vi "PixyCamSPI.vi"(11 "SPI Bus":T1) -> ()   [LabVIEW 2017]
doc: "This VI reads the bolcks identified by a PixyCam. It is designed within the FRC framework and is expected to be run on a RoboRIO using the SPI ports.\nThe slave select pins are used so several PixyCam can be used. \nRefer to http://cmucam.org/projects/cmucam5/wiki/Porting_Guide for wiring and code explanation\nUse PixyMon to define the protocol and signatures\n\n(c)2017 PY Le Bas"
uses:
  <vilib>/Rock Robotics/SystemInterfaces/spilib/spi_bus.ctl
  <vilib>/Rock Robotics/WPI/SPI/WPI_SPIMode.ctl
  Robot Global Data.vi
  <vilib>/Rock Robotics/Network Tables/NT Write Number.vi
panel:
  out "Blocks":T2(array[cluster])
  out "last frame data":u16[](array[numeric]) format="%.0x"
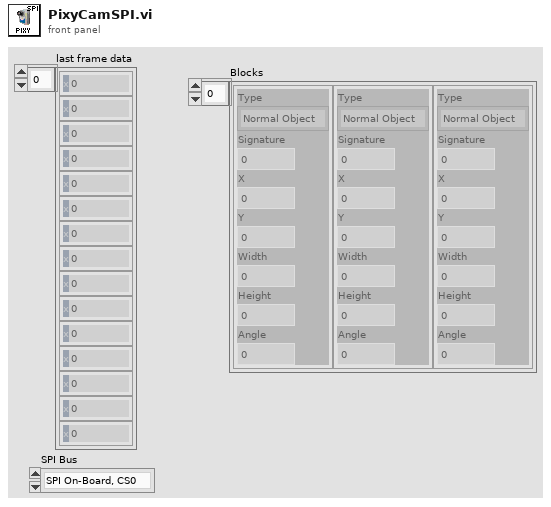
[diagram p1: front panel]
types:
  T1 = typedef "spi_bus.ctl" = enum16{"SPI On-Board, CS0", "SPI On-Board, CS1", "SPI On-Board, CS2", "SPI On-Board, CS3", "SPI MXP", "Invalid"}
  T2 = cluster{"Type":enum16{"Normal Object", "Color Object"}, "Signature":u16, "X":u16, "Y":u16, "Width":u16, "Height":u16, "Angle":u16}[]
  T3 = typedef "WPI_SPIMode.ctl" = enum16{"Mode 0 (Clk Idle Low,Sample on Leading)", "Mode 1 (Clk Idle Low,Sample on Trailing)", "Mode 2 (Clk Idle High,Sample on Leading)", "Mode 3 (Clk Idle High,Sample on Trailing)"}
  T4 = typedef "WPI_SPIDevRef.ctl" = cluster{"DevStatus":errorcluster, "Handle":i32, "SPI Bus":T1}
  T5 = cluster{"Type":enum16{"Normal Object", "Color Object"}, "Signature":u16, "X":u16, "Y":u16, "Width":u16, "Height":u16, "Angle":u16}
  T6 = cluster{"[0]":u16, "[1]":u16, "[2]":u16, "[3]":u16, "[4]":u16, "[5]":u16, "[6]":u16}
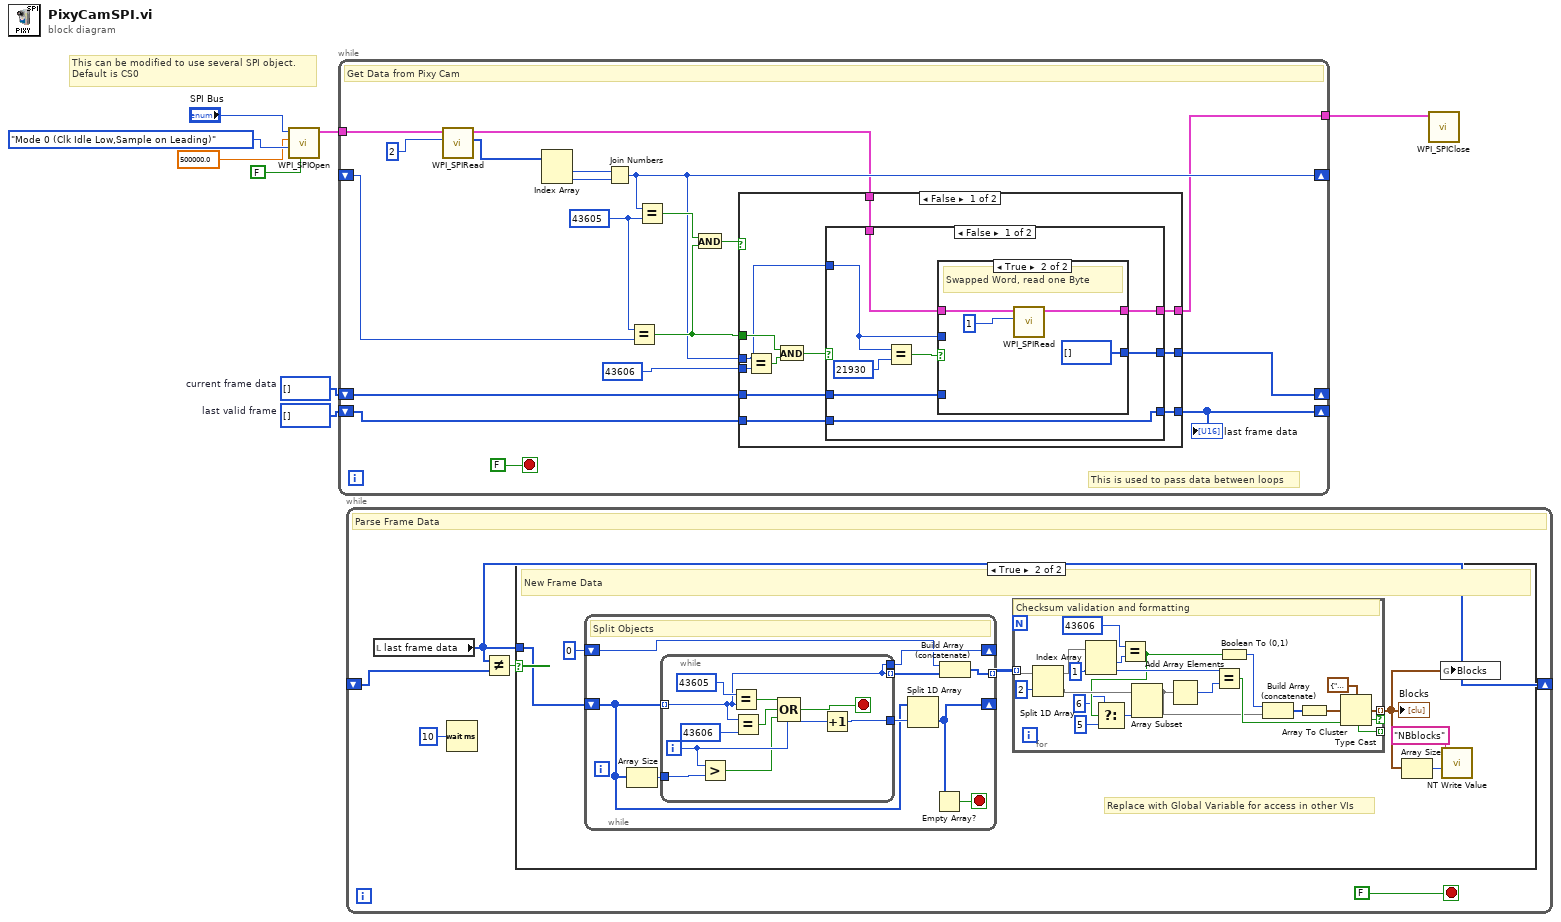
[diagram p0: block diagram]
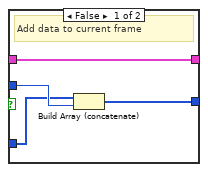
[diagram p3: hidden frame]
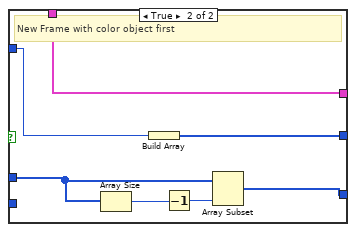
[diagram p4: hidden frame]
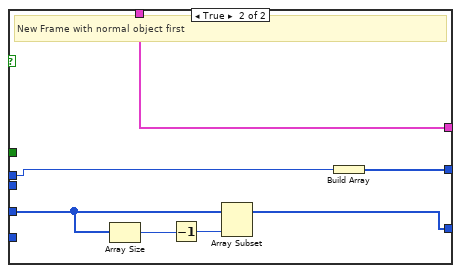
[diagram p5: hidden frame]
diagram:
  w5 = u16[] []  # current frame data
  w6 = u16[] []  # last valid frame
  # "This can be modified to use several SPI object.\nDefault is CS0"
  n1 = call <vilib>:"WPI_SPIOpen.vi"("Chip Select Active High (F)"=FALSE, "Mode (3)"=WPI_SPIMode."Mode 0 (Clk Idle Low,Sample on Leading)", "Clock Rate (Hz)"=500000.0, "SPI Bus"="SPI Bus") -> ("SPIDevRef"=w8:T4)  [unwired: 6 in, 1 out]
  n2 = while {
    tunnel: w8 -> [w27]
    tunnel: [w16] -> w7
    shift-right: [w18] -> _
    shift-left: _ -> [w23]
    shift-right: [w14] -> _
    shift-left: w5 -> [w15]
    shift-right: [w13] -> _
    shift-left: w6 -> [w12]
    stop <- FALSE stop-if-true
    w11 = u16 43605
    # "This is used to pass data between loops"
    # "Get Data from Pixy Cam"
    n3 = call <vilib>:"WPI_SPIRead.vi"("Num to Read"=2, "SPIDevRef"=w27) -> ("Received Data"=w26:u8[], "SPIDevRef"=w17:T4)  [unwired: 7 in, 1 out]
    n4 = Index Array(array=w26) -> (element #1=w25:u8, element #2=w24:u8)  [unwired: 2 in]
    n5 = Join Numbers(hi=w25, lo=w24) -> ((hi.lo)=w18:u16)
    n6 = Equal?(x=w11, y=w23) -> (x = y?=w20:bool)
    n7 = Equal?(x=w18, y=w11) -> (x = y?=w21:bool)
    n8 = And(x=w21, y=w20) -> (x .and. y?=w22:bool)
    n9 = case shown="False" w22 {
      tunnel: w20 -> [w38 _]
      tunnel: w18 -> [w28 w62]
      tunnel: u16 43606 -> [w36 _]
      tunnel: w17 -> [w34 w68]
      tunnel: [w33 w68] -> w16
      tunnel: w15 -> [w32 w65]
      tunnel: [w31 w63] -> w14
      tunnel: [w30 w67] -> w13
      tunnel: w12 -> [w29 _]
      frame False {
        n10 = Equal?(x=w28, y=w36) -> (x = y?=w37:bool)
        n11 = And(x=w38, y=w37) -> (x .and. y?=w35:bool)
        n12 = case shown="False" w35 {
          tunnel: w28 -> [w42 w56]
          tunnel: w34 -> [w45 w61]
          tunnel: [w44 w61] -> w33
          tunnel: w32 -> [w41 w58]
          tunnel: [w40 w55] -> w31
          tunnel: [w39 w57] -> w30
          tunnel: w29 -> [w39 _]
          frame False {
            n13 = Equal?(x=w42, y=u16 21930) -> (x = y?=w43:bool)
            n14 = case shown="True" w43 {
              tunnel: w45 -> [w50 w54]
              tunnel: [w50 w53] -> w44
              tunnel: w42 -> [w49 _]
              tunnel: w41 -> [w48 _]
              tunnel: [w47 u16[] []] -> w40
              frame False {
                # "Add data to current frame"
                n15 = Build Array (concatenate)(w48, w49) -> (w47:u16[])
              }
              frame True {
                # "Swapped Word, read one Byte"
                n16 = call <vilib>:"WPI_SPIRead.vi"("Num to Read"=1, "SPIDevRef"=w54) -> ("SPIDevRef"=w53:T4)  [unwired: 7 in, 2 out]
              }
            }
          }
          frame True {
            # "New Frame with color object first"
            n17 = Array Size(array=w58) -> (size(s)=w60:i32)
            n18 = Build Array(w56) -> (w55:u16[])
            n19 = Decrement(x=w60) -> (x-1=w59:i32)
            n20 = Array Subset(array=w58, length=w59) -> (w57:u16[])  [unwired: 1 in]
          }
        }
      }
      frame True {
        # "New Frame with normal object first"
        n21 = Array Size(array=w65) -> (size(s)=w66:i32)
        n22 = Decrement(x=w66) -> (x-1=w64:i32)
        n23 = Array Subset(array=w65, length=w64) -> (w67:u16[])  [unwired: 1 in]
        n24 = Build Array(w62) -> (w63:u16[])
      }
    }
    "last frame data" <- w13
  }
  n25 = while {
    shift-right: [w71] -> _
    shift-left: _ -> [w73]
    stop <- FALSE stop-if-true
    # "Parse Frame Data"
    n26 = local read "last frame data"() -> (w71:u16[])
    n27 = Wait (ms)(milliseconds to wait=u32 10) -> ()  [unwired: 1 out]
    n28 = Not Equal?(x=w71, y=w73) -> (x != y?=w72:bool)
    n29 = case shown="True" w72 {
      tunnel: w71 -> [_ w78]
      frame False {
        # "Same Frame"
      }
      frame True {
        # "Replace with Global Variable for access in other VIs"
        # "New Frame Data"
        n30 = while {
          shift-right: [w106] -> _
          shift-left: w78 -> [w104]
          tunnel: [w102] -> w77 mode=indexing
          shift-right: [w101] -> _
          shift-left: u16 0 -> [w100]
          stop <- w105 stop-if-true
          # "Split Objects"
          n31 = Array Size(array=w104) -> (size(s)=w103:i32)
          n32 = while {
            tunnel: w104 -> [w109] mode=indexing
            tunnel: [w109] -> w108 mode=indexing
            tunnel: [w114] -> w107
            tunnel: w103 -> [w112]
            tunnel: [w109] -> w101
            i -> [w111]
            stop <- w115 stop-if-true
            n33 = Greater?(x=w111, y=w112) -> (0:w110:bool)
            n34 = Equal?(x=u16 43605, y=w109) -> (x = y?=w117:bool)
            n35 = Equal?(x=w109, y=u16 43606) -> (x = y?=w116:bool)
            n36 = Compound Arithmetic op=OR(w117, w116, w110) -> (w115:bool)
            n37 = Increment(x=w111) -> (x+1=w114:i32)
          }
          n38 = Split 1D Array(array=w104, index=w107) -> (second subarray=w106:u16[])  [unwired: 1 out]
          n39 = Empty Array?(array=w106) -> (empty?=w105:bool)
          n40 = Build Array (concatenate)(w100, w108) -> (w102:u16[])
        }
        n41 = for {
          tunnel: w77 -> [w99] mode=indexing
          tunnel: [w88] -> w74 mode=indexing if=w86
          tunnel: [w86] -> _ mode=indexing
          # "Checksum validation and formatting"
          n42 = Split 1D Array(array=w99, index=2) -> (first subarray=w97:u16[], second subarray=w85:u16[])
          n43 = Index Array(array=w97, index #2=1 ("index")) -> (element #1=w91:u16, element #2=w96:u16)  [unwired: 1 in]
          n44 = Equal?(x=u16 43606, y=w91) -> (x = y?=w82:bool)
          n45 = Select(t=6 ("index"), s=w82, f=5 ("index")) -> (s? t:f=w83:i32)
          n46 = Array Subset(array=w85, length=w83) -> (w84:u16[])  [unwired: 1 in]
          n47 = Add Array Elements(numeric array=w84) -> (sum=w95:u16)
          n48 = Equal?(x=w96, y=w95) -> (x = y?=w86:bool)
          n49 = Boolean To (0,1)(Boolean=w82) -> (0, 1=w89:i16)
          n50 = Build Array (concatenate)(w89, w84) -> (w92:u16[])
          n51 = Array To Cluster(array=w92) -> (cluster=w93:T6)
          n52 = Type Cast(type=T5 {"Type"=enum."Color Object", "Signature"=1, "X"=100, "Y"=36, "Width"=50, "Height"=48, "Angle"=0} ("Blocks"), x=w93) -> (*(type *) &x=w88:T5)
        }
        "Blocks" <- w74
        n53 = Array Size(array=w74) -> (size(s)=w75:i32)
        n54 = global write "Robot Global Data.vi" "Blocks"(w74) -> ()
        n55 = call-poly <vilib>:"NT Write Value.vi"("Numeric"=w75, "Name"="NBblocks") -> ()  [unwired: 9 in, 1 out]
      }
    }
  }
  n56 = call <vilib>:"WPI_SPIClose.vi"("SPIDevRef"=w7) -> ()  [unwired: 10 in, 1 out]
